vi "sha256_pbkdf2.vi"(8 "dkLen (32octets=sha256)":i32=32, 9 "iterations":i32, 10 "salt":string, 11 "password":string) -> (3 "sha-256":u32[](array[numeric]) format="%08x")   [LabVIEW 2017, in "rpacini_hashlib.lvlib"]
doc: "RFC 2898C"
uses:
  rpacini_hashlib.lvlib
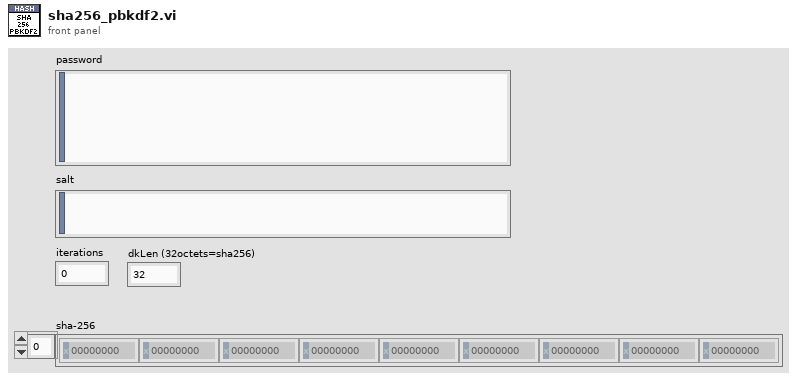
[diagram p1: front panel]
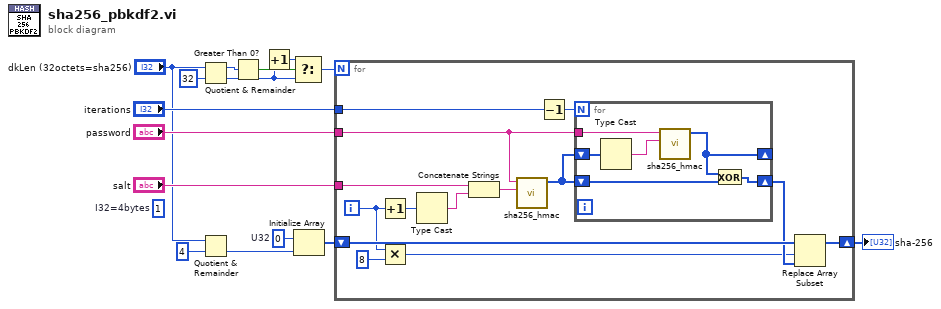
[diagram p0: block diagram]
diagram:
  w3 = u32 0  # U32
  (unwired) 1  # I32=4bytes
  n1 = Quotient & Remainder(x="dkLen (32octets=sha256)", y=32) -> (x-y*floor(x/y)=w11:i32, floor(x/y)=w9:i32)
  n2 = Quotient & Remainder(x="dkLen (32octets=sha256)", y=4) -> (floor(x/y)=w4:i32)  [unwired: 1 out]
  n3 = Greater Than 0?(x=w11) -> (x > 0?=w10:bool)
  n4 = Increment(x=w9) -> (x+1=w8:i32)
  n5 = Select(t=w8, s=w10, f=w9) -> (s? t:f=w7:i32)
  n6 = Initialize Array(w3, w4) -> (w2:u32[])
  n7 = for {
    N: w7 -> [_]
    tunnel: "iterations" -> [w29]
    tunnel: "salt" -> [w27]
    tunnel: "password" -> [w26]
    shift-right: [w20] -> w1
    shift-left: w2 -> [w21]
    i -> [w18]
    n8 = Increment(x=w18) -> (x+1=w22:i32)
    n9 = Multiply(x=w18, y=8) -> (x*y=w16:i32)
    n10 = Type Cast(x=w22) -> (*(type *) &x=w28:string)  [unwired: 1 in]
    n11 = Concatenate Strings(w27, w28) -> (w25:string)
    n12 = call "sha256_hmac.vi"("data"=w25, "key"=w26) -> ("sha256"=w23:u32[])  [unwired: 9 in]
    n13 = Decrement(x=w29) -> (x-1=w24:i32)
    n14 = for {
      N: w24 -> [_]
      tunnel: w26 -> [w35]
      shift-right: [w33] -> w19
      shift-left: w23 -> [w31]
      shift-right: [w32] -> _
      shift-left: w23 -> [w30]
      n15 = Type Cast(x=w30) -> (*(type *) &x=w34:string)  [unwired: 1 in]
      n16 = call "sha256_hmac.vi"("data"=w34, "key"=w35) -> ("sha256"=w32:u32[])  [unwired: 9 in]
      n17 = Exclusive Or(1:w31, 2:w32) -> (0:w33:u32[])
    }
    n18 = Replace Array Subset(array=w21, new element=w19, index=w16) -> (w20:u32[])
  }
  "sha-256" <- w1
